vi "Periodic Tasks.vi"(8 "error in":errorcluster) -> ()   [LabVIEW 2020]
doc: "This VI runs in parallel to other robot code. It can contain as many user-defined periodic loops as you need. These can carry out PID or other sorts of timed response."
uses:
  <vilib>/Rock Robotics/WPI/Utilities/WPI_GetSetVariantRefNum.vi
  Robot Global Data.vi
  <vilib>/Rock Robotics/Network Tables/NT Write Number.vi
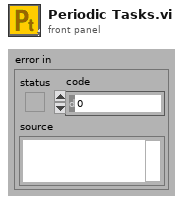
[diagram p1: front panel]
types:
  T1 = typedef "WPI_JoystickDevRef.ctl" = cluster{"Device":T2}
  T2 = typedef "WPI_JoystickDeviceEnum.ctl" = enum16{"USB 0", "USB 1", "USB 2", "USB 3", "USB 4", "USB 5"}
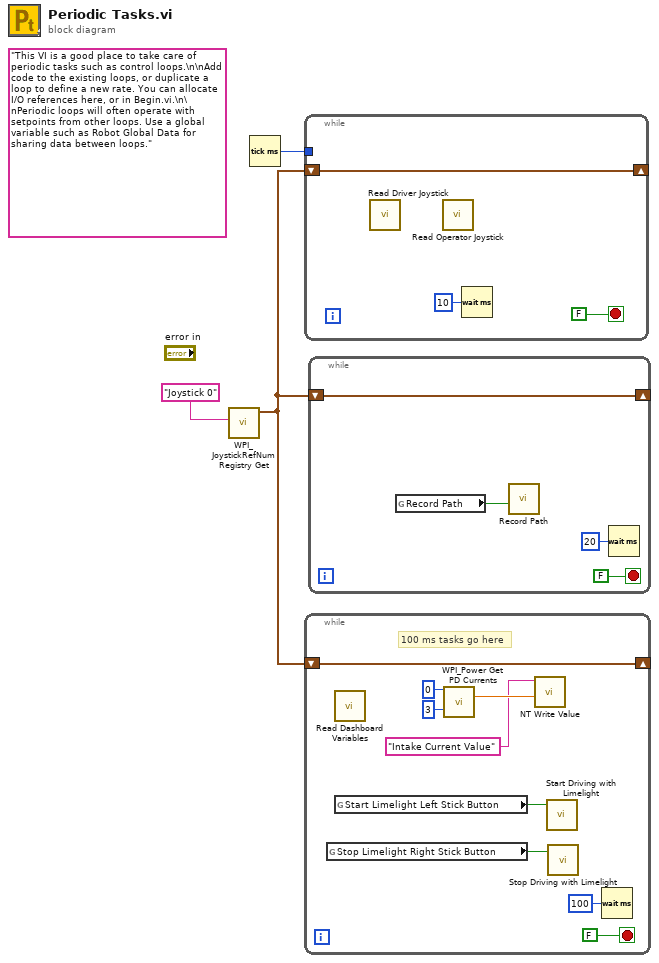
[diagram p0: block diagram]
diagram:
  (unwired) "This VI is a good place to take care of periodic tasks such as control loops.\n\nAdd code to the existing loops, or duplicate a loop to define a new rate. You can allocate I/O references here, or in Begin.vi.\n\nPeriodic loops will often operate with setpoints from other loops. Use a global variable such as Robot Global Data for sharing data between loops."
  n1 = call <vilib>:"WPI_JoystickRefNum Registry Get.vi"("refnum name"="Joystick 0") -> ("JoystickDevRef"=w1:T1)  [unwired: 1 in, 9 out]
  n2 = Tick Count (ms)() -> (millisecond timer value=w2:u32)
  n3 = while {
    shift-right: [w5] -> _
    shift-left: w1 -> [w5]
    tunnel: w2 -> [_]
    stop <- FALSE stop-if-true
    n4 = call "Read Driver Joystick.vi"() -> ()  [unwired: 12 in]
    n5 = call "Read Operator Joystick.vi"() -> ()  [unwired: 12 in]
    n6 = Wait (ms)(milliseconds to wait=u32 10) -> ()  [unwired: 1 out]
  }
  n7 = while {
    shift-right: [w13] -> _
    shift-left: w1 -> [w13]
    stop <- FALSE stop-if-true
    # "100 ms tasks go here"
    n8 = global read "Robot Global Data.vi" "Stop Limelight Right Stick Button"() -> (w7:bool)
    n9 = call "Read Dashboard Variables.vi"() -> ()  [unwired: 12 in]
    n10 = global read "Robot Global Data.vi" "Start Limelight Left Stick Button"() -> (w8:bool)
    n11 = call <vilib>:"WPI_Power Get PD Currents.vi"("Power Distribution (def)"=u8 0, "PD Channel"=3) -> ("current (A)"=w10:dbl)  [unwired: 10 in, 3 out]
    n12 = call-poly <vilib>:"NT Write Value.vi"("Numeric"=w10, "Name"="Intake Current Value") -> ()  [unwired: 9 in, 1 out]
    n13 = call "Start Driving with Limelight.vi"("Drive with Limelight"=w8) -> ()  [unwired: 11 in]
    n14 = call "Stop Driving with Limelight.vi"("Drive with Limelight"=w7) -> ()  [unwired: 11 in]
    n15 = Wait (ms)(milliseconds to wait=u32 100) -> ()  [unwired: 1 out]
  }
  n16 = while {
    shift-right: [w16] -> _
    shift-left: w1 -> [w16]
    stop <- FALSE stop-if-true
    n17 = global read "Robot Global Data.vi" "Record Path"() -> (w17:bool)
    n18 = call "Record Path.vi"("Record Path"=w17) -> ()  [unwired: 11 in]
    n19 = Wait (ms)(milliseconds to wait=u32 20) -> ()  [unwired: 1 out]
  }
